vi "Div.vi"(10 "B":dbl, 11 "A":dbl) -> (3 "C":dbl)   [LabVIEW 2018]
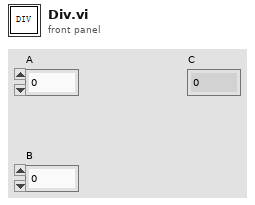
[diagram p1: front panel]
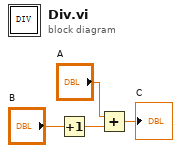
[diagram p0: block diagram]
diagram:
  n1 = Increment(x="B") -> (x+1=w2:dbl)
  n2 = Add(x="A", y=w2) -> (x+y=→"C":dbl)
